vi "call library test.vi"() -> ()   [LabVIEW 2023]
uses:
  cx-labview-wrapper/build/x64/Release/cx-labview-wrapper.dll
  CX Labview Wrapper.lvlib
  <vilib>/DLR/CMH Lib/Message Queue.lvlib
  <vilib>/DLR/CMH Lib/Message Queue/Enqueue Message.vi
panel:
  out "response":string
  out "index of not equal element":i32
  out "success write":i32
  out "success pcd write":i32
  in  "stop":bool
  out "Read Tif":u16[][](graph)
  in  "error in (no error)":errorcluster
  out "success read":i32
  out "error out":errorcluster
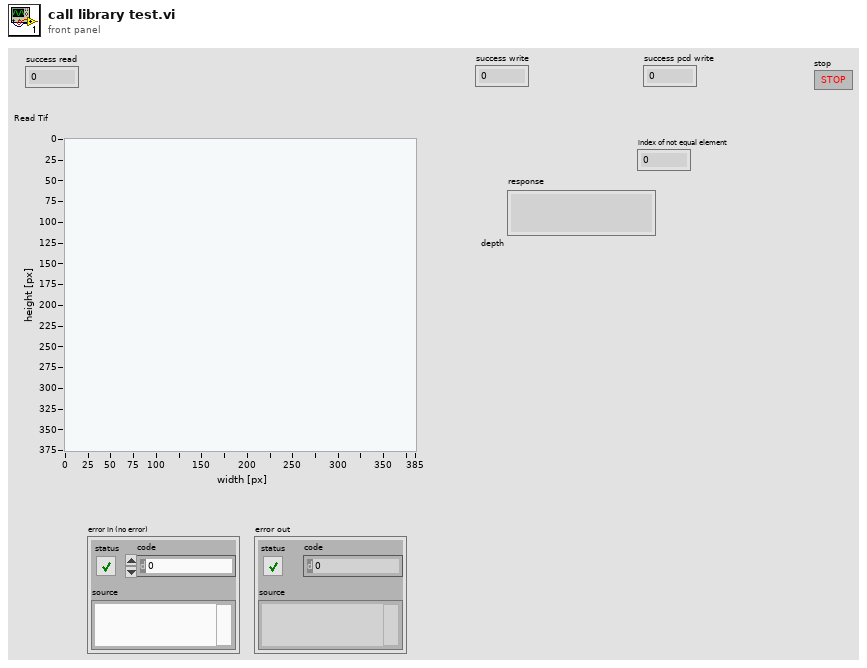
[diagram p1: front panel]
types:
  T1 = typedef "Messenger-t'Message Queue.lvlib-Message Cluster.ctl'.lvlib/))Channel.ctl" = refnum<queue>
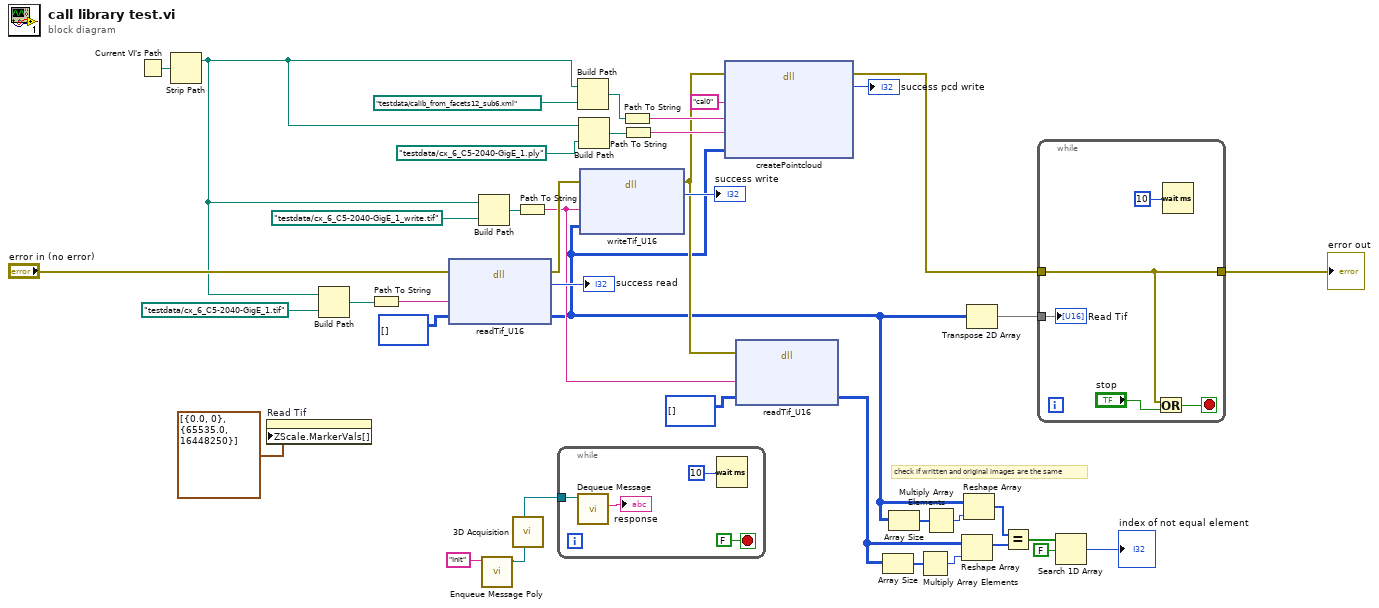
[diagram p0: block diagram]
diagram:
  # "check if written and original images are the same"
  n1 = Current VI's Path() -> (path=w31:path)
  n2 = Strip Path(path=w31) -> (stripped path=w21:path)  [unwired: 1 out]
  n3 = property on="Read Tif" class="IntGraph (strict)"("ZScale.MarkerVals[]"=cluster{dbl, u32}[] [{0.0, 0}, {65535.0, 16448250}] ("Z Scale.Marker Values[]")) -> ()  [unwired: 2 in, 2 out]
  n4 = Build Path(base path=w21, name or relative path=path "testdata/cx_6_C5-2040-GigE_1.tif") -> (appended path=w33:path)
  n5 = Path To String(path=w33) -> (string=w35:string)
  n6 = dll-call lib="D:/git/CX-LabVIEW-Wrapper/cx-labview-wrapper/build/x64/Release/cx-labview-wrapper.dll" fn="readTif_U16"(error in="error in (no error)", "fname"=w35, "rangeImg"=u16[][] []) -> (error out=w23:errorcluster, "success"=→"success read":i32, "rangeImg"=w4:u16[][])  [unwired: 3 in, 1 out]
  n7 = Build Path(base path=w21, name or relative path=path "testdata/cx_6_C5-2040-GigE_1_write.tif") -> (appended path=w20:path)
  n8 = call-poly <vilib>:"Enqueue Message Poly.vi"("Message"="Init") -> ("channel"=w3:T1)  [unwired: 10 in]
  n9 = call "3D Acquisition.vi"("remote cmd"=w3) -> ("remote response"=w1:T1)  [unwired: 10 in]
  n10 = Path To String(path=w20) -> (string=w15:string)
  n11 = while {
    tunnel: w1 -> [w45]
    stop <- FALSE stop-if-true
    n12 = call <vilib>:"Dequeue Message.vi"("channel"=w45) -> ("message"=→"response":string)  [unwired: 8 in, 2 out]
    n13 = Wait (ms)(milliseconds to wait=u32 10) -> ()  [unwired: 1 out]
  }
  n14 = Build Path(base path=w21, name or relative path=path "testdata/calib_from_facets12_sub6.xml") -> (appended path=w25:path)
  n15 = Build Path(base path=w21, name or relative path=path "testdata/cx_6_C5-2040-GigE_1.ply") -> (appended path=w29:path)
  n16 = dll-call lib="D:/git/CX-LabVIEW-Wrapper/cx-labview-wrapper/build/x64/Release/cx-labview-wrapper.dll" fn="writeTif_U16"(error in=w23, "fname"=w15, "rangeImg"=w4) -> (error out=w16:errorcluster, "success"=→"success write":i32)  [unwired: 4 in, 1 out]
  n17 = Path To String(path=w25) -> (string=w24:string)
  n18 = Path To String(path=w29) -> (string=w28:string)
  n19 = dll-call lib="D:/git/CX-LabVIEW-Wrapper/cx-labview-wrapper/build/x64/Release/cx-labview-wrapper.dll" fn="createPointcloud"(error in=w16, "calibId"="cal0", "calibFile"=w24, "pcdFile"=w28, "rangeImg"=w4) -> (error out=w36:errorcluster, "success"=→"success pcd write":i32)  [unwired: 6 in, 1 out]
  n20 = dll-call lib="D:/git/CX-LabVIEW-Wrapper/cx-labview-wrapper/build/x64/Release/cx-labview-wrapper.dll" fn="readTif_U16"(error in=w16, "fname"=w15, "rangeImg"=u16[][] []) -> ("rangeImg"=w9:u16[][])  [unwired: 4 in, 2 out]
  n21 = Array Size(array=w9) -> (size(s)=w8:i32[])
  n22 = Array Size(array=w4) -> (size(s)=w6:i32[])
  n23 = Multiply Array Elements(1:w8) -> (0:w7:i32)
  n24 = Multiply Array Elements(1:w6) -> (0:w5:i32)
  n25 = Reshape Array(w9, w7) -> (w14:u16[])
  n26 = Reshape Array(w4, w5) -> (w13:u16[])
  n27 = Transpose 2D Array(2D array=w4) -> (transposed array=w39:u16[][])
  n28 = Equal?(x=w13, y=w14) -> (x = y?=w12:bool[])
  n29 = while {
    tunnel: w39 -> [w50]
    tunnel: w36 -> [w46]
    tunnel: [w46] -> w38
    stop <- w48 stop-if-true
    n30 = Or(x=w46, y="stop") -> (x .or. y?=w48:bool)
    n31 = Wait (ms)(milliseconds to wait=u32 10) -> ()  [unwired: 1 out]
    "Read Tif" <- w50
  }
  "error out" <- w38
  n32 = Search 1D Array(1D array=w12, element=FALSE) -> (index of element=→"index of not equal element":i32)  [unwired: 1 in]
